vi "depositsubvi.vi"(11 "Enter the Amount":dbl) -> (3 "Numeric":dbl)   [LabVIEW 2012]
uses:
  Globalvariable.vi
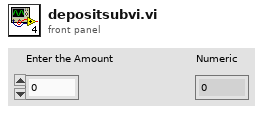
[diagram p1: front panel]
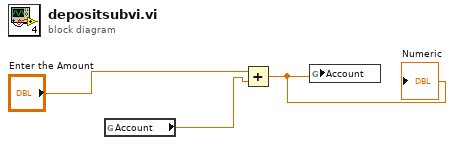
[diagram p0: block diagram]
diagram:
  n1 = global read "Globalvariable.vi" "Account"() -> (w1:dbl)
  n2 = Add(x="Enter the Amount", y=w1) -> (x+y=w3:dbl)
  "Numeric" <- w3
  n3 = global write "Globalvariable.vi" "Account"(w3) -> ()
